vi "Disconnect Core.vi"(8 "error in (no error)":errorcluster, 11 "DIMConnection in":refnum<class "DIMConnection.lvclass">) -> (0 "error out":errorcluster, 3 "DIMConnection out":refnum<class "DIMConnection.lvclass">)   [LabVIEW 2014, in "CS++DIM.lvlib" / "DIMConnection.lvclass"]
doc: "Opene reference to a process variable."
uses:
  DIMConnection.lvclass
  DimLVEvent/LVDimInterface/LVDimInterface.lvlib
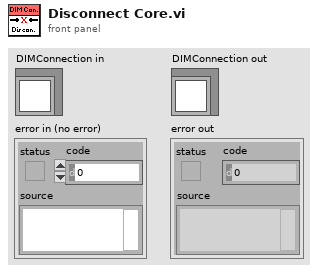
[diagram p1: front panel]
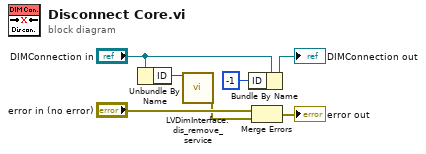
[diagram p0: block diagram]
diagram:
  n1 = Unbundle By Name("DIMConnection in") -> ("ID"=w7:i32)
  n2 = call "LVDimInterface.dis_remove_service.vi"("my_serviceID"=w7) -> ("error out"=w5:errorcluster)  [unwired: 18 in]
  n3 = Bundle By Name(cluster="DIMConnection in", "ID"=-1) -> (→"DIMConnection out":refnum<class "DIMConnection.lvclass">)
  n4 = Merge Errors("error in (no error)", w5) -> (→"error out":errorcluster)
